vi "Modify Client Controls.vi"(6 "default_value":variant, 8 "error in":errorcluster, 9 "control name":string, 10 "parameter data":T1[](array[typedef]), 11 "vi refnum":refnum<vi>) -> (0 "error out":errorcluster)   [LabVIEW 2021, in "MeasurementClient Editor.lvlib"]
uses:
  MeasurementClient Editor.lvlib
  <vilib>/gRPC/Generated APIs/ni/measurementlink/measurement/v2/Measurement Service Client V2/RPC Messages/ni_measurementlink_measurement_v2_ConfigurationParameter.ctl
  <vilib>/gRPC/Generated APIs/ni/measurementlink/measurement/v2/Measurement Service Client V2/RPC Messages/google_protobuf_Field_Kind.ctl
  <vilib>/gRPC/Generated APIs/ni/measurementlink/measurement/v2/Measurement Service Client V2/RPC Messages/ni_measurementlink_measurement_v2_ConfigurationParameter_AnnotationsEntry.ctl
  <vilib>/Utility/miscctls.llb/LVPositionTypeDef.ctl
  <vilib>/gRPC/Generated APIs/ni/measurementlink/measurement/v2/Measurement Service Client V2/Measurement Service Client V2.lvlib
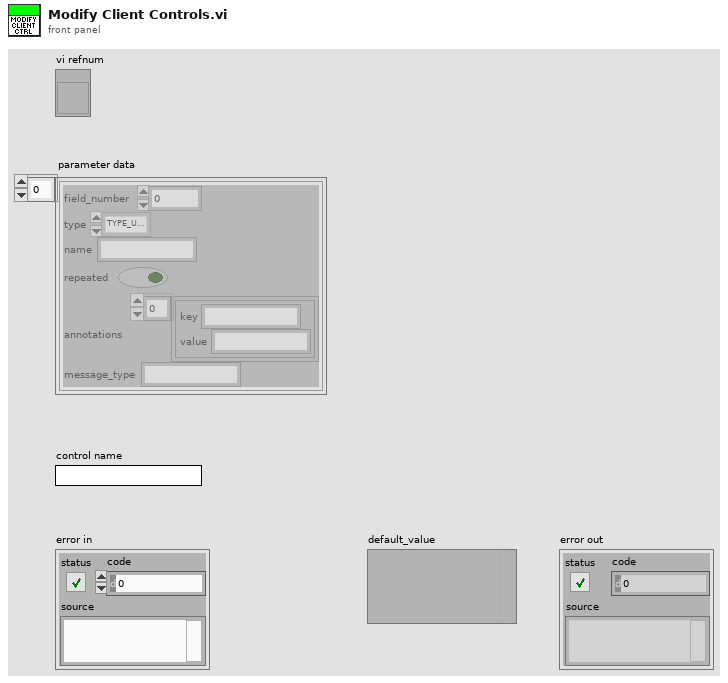
[diagram p1: front panel]
types:
  T1 = typedef "Measurement Service Client V2.lvlib/ni_measurementlink_measurement_v2_ConfigurationParameter.ctl" = cluster{"field_number":i32, "type":T2, "name":string, "repeated":bool, "annotations":T3[], "message_type":string}
  T2 = typedef "Measurement Service Client V2.lvlib/google_protobuf_Field_Kind.ctl" = enum32{"TYPE_UNKNOWN", "TYPE_DOUBLE", "TYPE_FLOAT", "TYPE_INT64", "TYPE_UINT64", "TYPE_INT32", "TYPE_FIXED64", "TYPE_FIXED32", "TYPE_BOOL", "TYPE_STRING", "TYPE_GROUP", "TYPE_MESSAGE", "TYPE_BYTES", "TYPE_UINT32", "TYPE_ENUM", "TYPE_SFIXED32", "TYPE_SFIXED64", "TYPE_SINT32", "TYPE_SINT64"}
  T3 = typedef "Measurement Service Client V2.lvlib/ni_measurementlink_measurement_v2_ConfigurationParameter_AnnotationsEntry.ctl" = cluster{"key":string, "value":string}
  T4 = typedef "LVPositionTypeDef.ctl" = cluster{"Left":i32, "Top":i32}
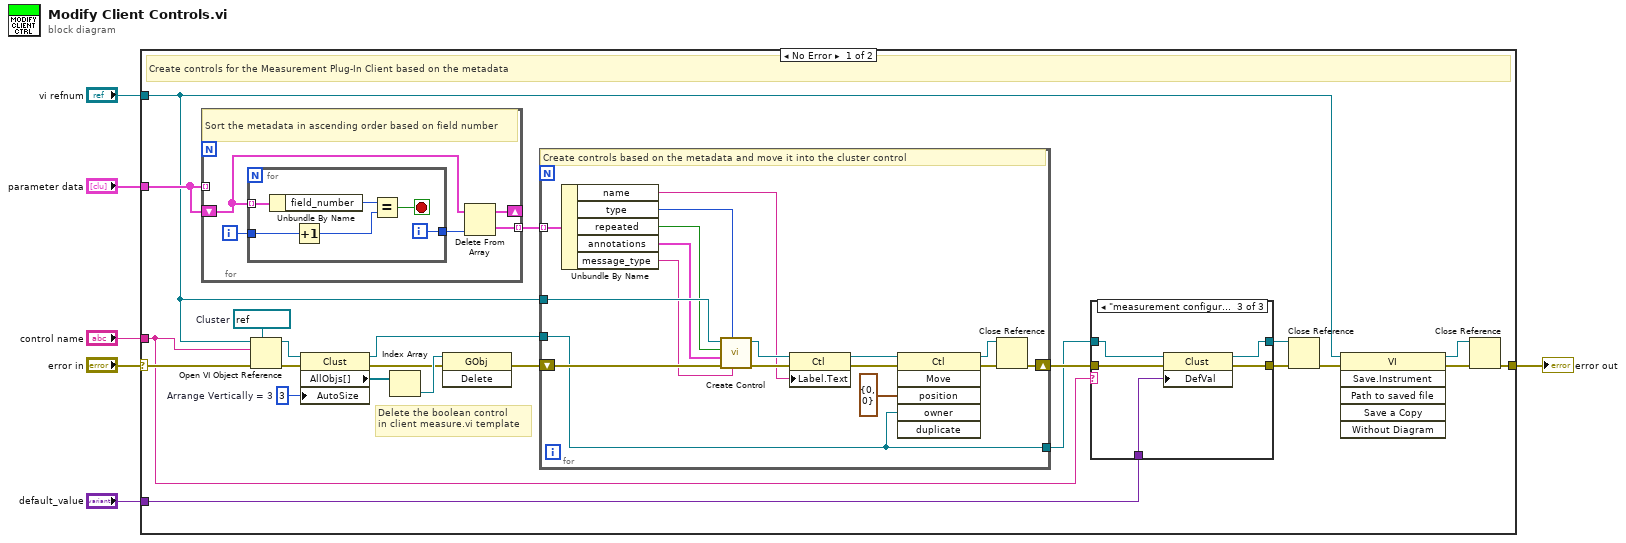
[diagram p0: block diagram]
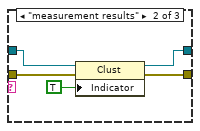
[diagram p3: hidden frame]
diagram:
  n1 = case shown="No Error" "error in" {
    selector: "error in" -> [w23 w70]
    tunnel: "control name" -> [w15 _]
    tunnel: "parameter data" -> [w13 _]
    tunnel: "vi refnum" -> [w10 _]
    tunnel: [w8 w70] -> w3
    tunnel: "default_value" -> [w7 _]
    frame No Error {
      w22 = u32 3  # Arrange Vertically = 3
      w29 = refnum<vi> refnum  # Cluster
      # "Delete the boolean control\nin client measure.vi template"
      # "Create controls for the Measurement Plug-In Client based on the metadata"
      n2 = for {
        shift-right: [w60] -> _
        shift-left: w13 -> [w61]
        tunnel: [w59] -> w14 mode=indexing
        tunnel: w13 -> [_] mode=indexing
        i -> [w63]
        # "Sort the metadata in ascending order based on field number"
        n3 = for {
          tunnel: w61 -> [w66] mode=indexing
          tunnel: w63 -> [w69]
          tunnel: [w65] -> w62
          i -> [w65]
          stop <- w64 stop-if-true
          n4 = Unbundle By Name(w66) -> ("field_number"=w68:i32)
          n5 = Increment(x=w69) -> (x+1=w67:i32)
          n6 = Equal?(x=w68, y=w67) -> (x = y?=w64:bool)
        }
        n7 = Delete From Array(array=w61, index=w62) -> (deleted portion=w59:T1, array with subset deleted=w60:T1[])  [unwired: 1 in]
      }
      n8 = Open VI Object Reference(7:w29, 8:w23, 10:w15, 11:w10) -> (0:w27:errorcluster, 3:w28:refnum<vi>)
      n9 = property class="Clust"(reference=w28, error in=w27, "AutoSize"=w22) -> (reference out=w19:refnum<vi>, error out=w24:errorcluster, "AllObjs[]"=w26:refnum<vi>[])
      n10 = Index Array(array=w26) -> (element=w25:refnum<vi>)  [unwired: 1 in]
      n11 = invoke class="GObj" method="Delete"(reference=w25, error in=w24) -> (error out=w21:errorcluster)  [unwired: 1 in, 2 out]
      n12 = for {
        shift-right: [w46] -> w20
        shift-left: w21 -> [w58]
        tunnel: w10 -> [w56]
        tunnel: w19 -> [w44]
        tunnel: [w44] -> w17
        tunnel: w14 -> [w42] mode=indexing
        # "Create controls based on the metadata and move it into the cluster control"
        n13 = Unbundle By Name(w42) -> ("name"=w50:string, "type"=w54:T2, "repeated"=w55:bool, "annotations"=w53:T3[], "message_type"=w52:string)
        n14 = call "Create Control.vi"("message_type"=w52, "type"=w54, "error in"=w58, "annotations"=w53, "is repeated?"=w55, "vi refnum"=w56) -> ("error out"=w57:errorcluster, "control ref"=w51:refnum<vi>)  [unwired: 4 in]
        n15 = property class="Ctl"(reference=w51, error in=w57, "Label.Text"=w50) -> (reference out=w49:refnum<vi>, error out=w48:errorcluster)
        n16 = invoke class="Ctl" method="Move"(reference=w49, error in=w48, "position"=T4 {"Left"=0, "Top"=0}, "owner"=w44) -> (reference out=w45:refnum<vi>, error out=w47:errorcluster)  [unwired: 2 in, 4 out]
        n17 = Close Reference(reference=w45, error in (no error)=w47) -> (error out=w46:errorcluster)
      }
      n18 = case shown="\"measurement configuration\"" w15 {
        tunnel: w20 -> [w31 w36 w41]
        tunnel: [w31 w35 w40] -> w18
        tunnel: w17 -> [w30 w34 w39]
        tunnel: [w30 w33 w38] -> w16
        tunnel: w7 -> [_ _ w37]
        frame Default {
        }
        frame "measurement results" {
          n19 = property class="Clust"(reference=w34, error in=w36, "Indicator"=TRUE) -> (reference out=w33:refnum<vi>, error out=w35:errorcluster)
        }
        frame "measurement configuration" {
          n20 = property class="Clust"(reference=w39, error in=w41, "DefVal"=w37) -> (reference out=w38:refnum<vi>, error out=w40:errorcluster)
        }
      }
      n21 = Close Reference(reference=w16, error in (no error)=w18) -> (error out=w9:errorcluster)
      n22 = invoke class="VI" method="Save.Instrument"(reference=w10, error in=w9) -> (reference out=w12:refnum<vi>, error out=w11:errorcluster)  [unwired: 4 in, 4 out]
      n23 = Close Reference(reference=w12, error in (no error)=w11) -> (error out=w8:errorcluster)
    }
    frame Error {
      # "Pass"
    }
  }
  "error out" <- w3
